vi "Configure Third Order Intercept.vi"   [LabVIEW 2020, in "Anritsu Signal Analyzer Series.lvlib"]
doc: "Configure the TOI measurment settings of the spectrum analyzer."
uses:
  Anritsu Signal Analyzer Series.lvlib
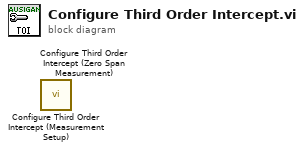
[diagram p0: block diagram]
diagram:
  n1 = call "Configure Third Order Intercept (Measurement Setup).vi"() -> ()  [unwired: 14 in, 2 out]
  n2 = call "Configure Third Order Intercept (Zero Span Measurement).vi"() -> ()  [unwired: 14 in, 2 out]
